vi "Acroname_Port_Enable.vi"(8 "error in (no error)":errorcluster, 9 "Current Max Amps limit (1.2)":dbl=1.2 format="%#_13g", 11 "Port Number":i32) -> (0 "error out":errorcluster, 1 "Max Current (µA)":u32, 2 "Min Voltage (µV)":u32, 3 "Enable Successful?":bool)   [LabVIEW 2025]
uses:
  1b1786e0-183b-4c19-b690-1d9e1fdb2131.vi
  27beaf38-548c-40ef-8c97-2fa24fe30fbd.vi
  31bf49dc-6773-40db-bb53-a572b45535a5.vi
  BrainStem2_LabVIEW_Library.lvlib
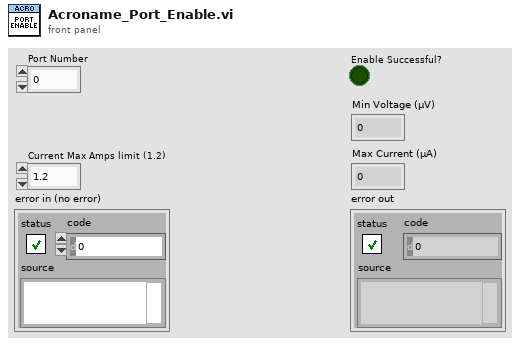
[diagram p1: front panel]
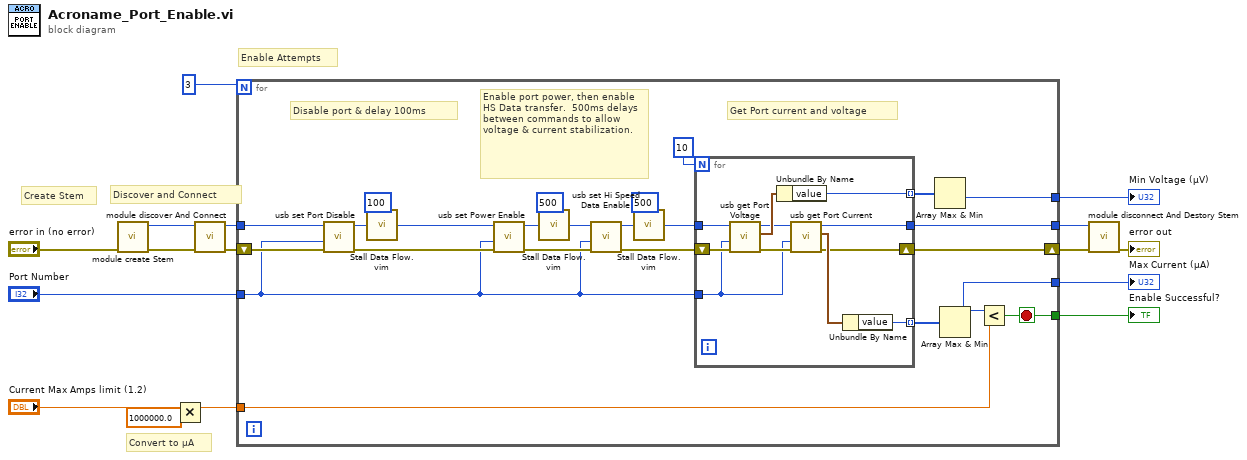
[diagram p0: block diagram]
diagram:
  # "Convert to µA"
  # "Discover and Connect"
  # "Create Stem"
  # "Enable Attempts"
  n1 = call "module create Stem.vi"("error in (no error)"="error in (no error)") -> ("error out"=w11:errorcluster, "id out"=w16:u32)  [unwired: 8 in, 1 out]
  n2 = Multiply(x="Current Max Amps limit (1.2)", y=1000000.0) -> (x*y=w2:dbl)
  n3 = call "module discover And Connect.vi"("error in (no error)"=w11, "id"=w16) -> ("error out"=w10:errorcluster, "id out"=w15:u32)  [unwired: 7 in, 1 out]
  n4 = for {
    N: 3 -> [_]
    tunnel: w15 -> [w40]
    tunnel: [w38] -> w14
    tunnel: "Port Number" -> [w24]
    tunnel: w2 -> [w21]
    shift-right: [w20] -> w7
    shift-left: w10 -> [w35]
    tunnel: [w19] -> w5
    tunnel: [w18] -> w4
    tunnel: [w17] -> w3
    stop <- w19 stop-if-true
    # "Get Port current and voltage"
    # "Enable port power, then enable HS Data transfer.  500ms delays between commands to allow voltage & current stabilization."
    # "Disable port & delay 100ms"
    n5 = call "usb set Port Disable.vi"("error in (no error)"=w35, "channel"=w24, "id"=w40) -> ("error out"=w33:errorcluster, "id out"=w37:u32)  [unwired: 6 in, 1 out]
    n6 = call "Stall Data Flow.vim"("value in"=w37, "milliseconds to wait"=100) -> ("value out"=w34:u32)  [unwired: 1 out]
    n7 = call "usb set Power Enable.vi"("error in (no error)"=w33, "channel"=w24, "id"=w34) -> ("error out"=w29:errorcluster, "id out"=w31:u32)  [unwired: 6 in, 1 out]
    n8 = call "Stall Data Flow.vim"("value in"=w31, "milliseconds to wait"=500) -> ("value out"=w30:u32)  [unwired: 1 out]
    n9 = call "usb set Hi Speed Data Enable.vi"("error in (no error)"=w29, "channel"=w24, "id"=w30) -> ("error out"=w25:errorcluster, "id out"=w27:u32)  [unwired: 6 in, 1 out]
    n10 = call "Stall Data Flow.vim"("value in"=w27, "milliseconds to wait"=500) -> ("value out"=w26:u32)  [unwired: 1 out]
    n11 = for {
      N: 10 -> [_]
      tunnel: w26 -> [w48]
      tunnel: [w47] -> w38
      tunnel: w24 -> [w44]
      shift-right: [w43] -> w20
      shift-left: w25 -> [w46]
      tunnel: [w42] -> w23 mode=indexing
      tunnel: [w41] -> w22 mode=indexing
      n12 = call "usb get Port Voltage.vi"("error in (no error)"=w46, "channel"=w44, "id"=w48) -> ("error out"=w45:errorcluster, "result out"=w51:cluster{"value":i32, "error":i32}, "id out"=w49:u32)  [unwired: 6 in]
      n13 = Unbundle By Name(w51) -> ("value"=w42:i32)
      n14 = call "usb get Port Current.vi"("error in (no error)"=w45, "channel"=w44, "id"=w49) -> ("error out"=w43:errorcluster, "result out"=w50:cluster{"value":i32, "error":i32}, "id out"=w47:u32)  [unwired: 6 in]
      n15 = Unbundle By Name(w50) -> ("value"=w41:i32)
    }
    n16 = Array Max & Min(array=w23) -> (min value=w17:i32)  [unwired: 3 out]
    n17 = Array Max & Min(array=w22) -> (max value=w18:i32)  [unwired: 3 out]
    n18 = Less?(x=w18, y=w21) -> (x < y?=w19:bool)
  }
  "Enable Successful?" <- w5
  "Max Current (µA)" <- w4
  "Min Voltage (µV)" <- w3
  n19 = call "module disconnect And Destory Stem.vi"("error in (no error)"=w7, "id"=w14) -> ("error out"=→"error out":errorcluster)  [unwired: 7 in, 2 out]
